vi "Set Port Status.vi"(8 "error in (no error)":errorcluster, 9 "Value":string, 10 "Port":dbl, 11 "object in":refnum<class "TI.lvclass">) -> (0 "error out":errorcluster, 3 "object out":refnum<class "TI.lvclass">)   [LabVIEW 2020, in "TI.lvclass"]
uses:
  TI.lvclass
  TI.lvclass/TI.ctl
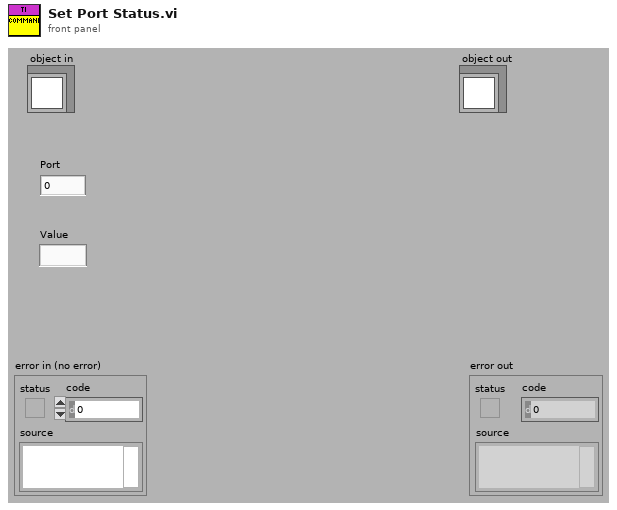
[diagram p1: front panel]
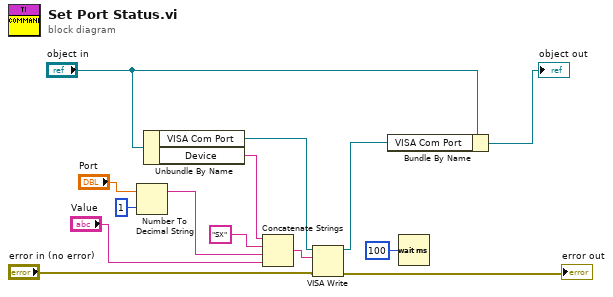
[diagram p0: block diagram]
diagram:
  n1 = Number To Decimal String(number="Port", width (-)=i16 1) -> (decimal integer string=w12:string)
  n2 = Unbundle By Name("object in") -> ("VISA Com Port"=w6:refnum<visa-resource-name>, "Device"=w7:string)
  n3 = Concatenate Strings(w7, "SX" ("string"), w12, "Value") -> (w14:string)
  n4 = VISA Write(VISA resource name=w6, write buffer=w14, error in (no error)="error in (no error)") -> (VISA resource name out=w11:refnum<visa-resource-name>, error out=→"error out":errorcluster)  [unwired: 1 out]
  n5 = Bundle By Name(cluster="object in", "VISA Com Port"=w11) -> (→"object out":refnum<class "TI.lvclass">)
  n6 = Wait (ms)(milliseconds to wait=u32 100) -> ()  [unwired: 1 out]
